vi "debug.vi"(8 "error in (no error)":errorcluster, 9 "ms update rate (1000)":u32=1000) -> (0 "error out":errorcluster, 3 "debug":string)   [LabVIEW 2017, in "rethinkdb.lvlib"]
uses:
  rethinkdb.lvlib
  debug_action.ctl
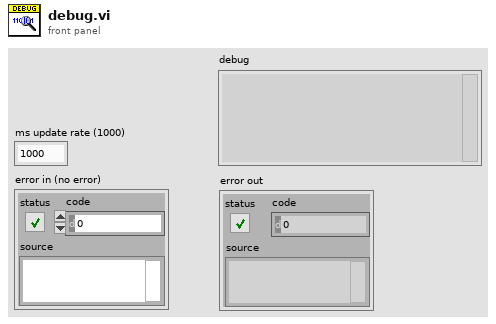
[diagram p1: front panel]
types:
  T1 = typedef "rethinkdb.lvlib/debug_action.ctl" = enum8{"get", "set_query", "set_response", "clear"}
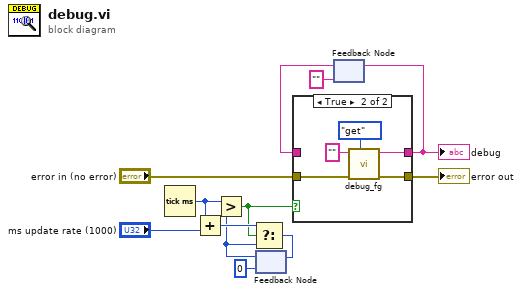
[diagram p0: block diagram]
diagram:
  n1 = Tick Count (ms)() -> (millisecond timer value=w8:u32)
  n2 = Add(x=w8, y="ms update rate (1000)") -> (x+y=w7:u32)
  n3 = feedback #1(u32 0) -> (w6:u32)
  n4 = Greater?(x=w8, y=w6) -> (0:w4:bool)
  n5 = Select(t=w7, s=w4, f=w6) -> (s? t:f=w5:u32)
  n6 = feedback-in #1(w5) -> ()
  n7 = feedback #2("") -> (w2:string)
  n8 = case shown="True" w4 {
    tunnel: "error in (no error)" -> [w13 w19]
    tunnel: [w13 w18] -> w11
    tunnel: [w14 w15] -> w9
    tunnel: w2 -> [w14 _]
    frame False {
    }
    frame True {
      n9 = call "debug_fg.vi"("action"=debug_action."get", "error in (no error)"=w19, "data"="") -> ("error out"=w18:errorcluster, "debug"=w15:string)  [unwired: 7 in]
    }
  }
  "error out" <- w11
  "debug" <- w9
  n10 = feedback-in #2(w9) -> ()
